vi "proiectu fara drona.vi"() -> ()   [LabVIEW 2015]
uses:
  globala.vi
  lee_3/bin/Debug/lee_3.dll
  BmpWork/lee_4/bin/Debug/lee_4.dll
panel:
  out "Numeric":dbl
  out "Image 2":T1(plugin-control)
  out "Image":T1(plugin-control)
  out "Computing Path":bool
  out "Finding START/STOP":bool
  out "Creating image from matrix":bool
  out "Started stitching":bool
  out "Started normalising and cutting":bool
  out "Curently at image":string
  out "return type 2":i32
  out "return type":i32
  in  "Numar de Poze":i32
  in  "Path to template":path
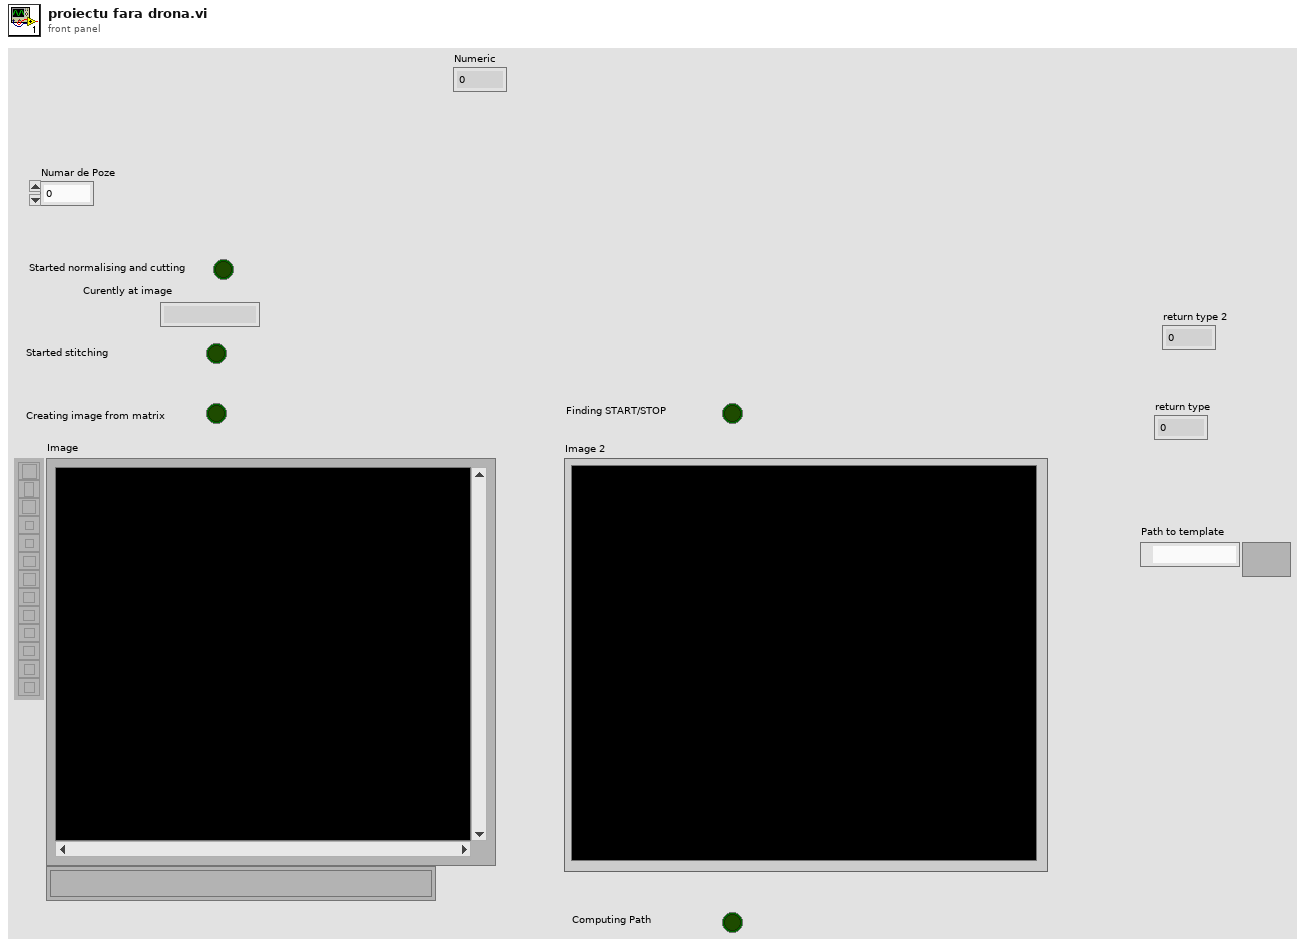
[diagram p1: front panel]
types:
  T1 = typedef "IMAQ Image.ctl" = refnum<image>
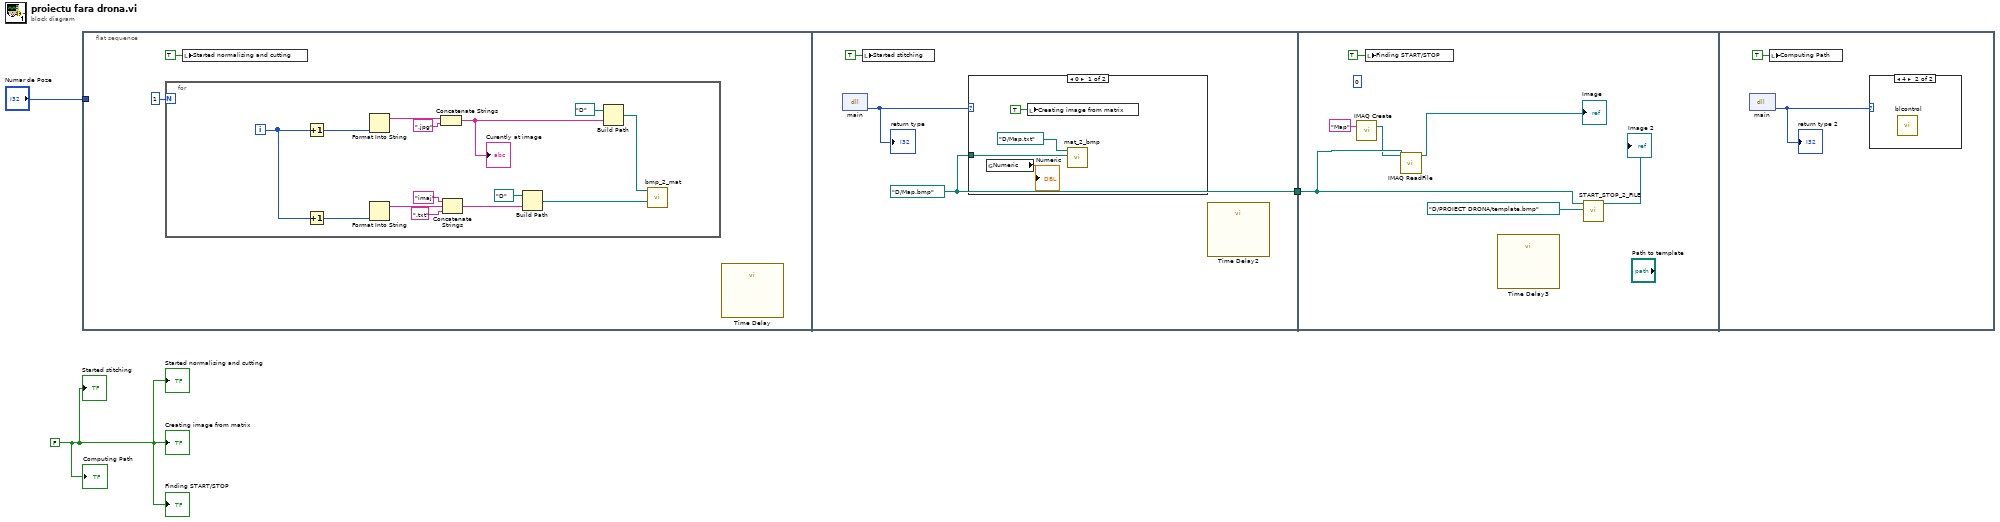
[diagram p0: block diagram]
diagram:
  w1 = FALSE
  n1 = flat-sequence {
    tunnel: "Numar de Poze" -> [_]
    tunnel: [w21] -> w3
    tunnel: w3 -> [w30]
    frame #0 {
      n2 = for {
        N: 1 -> [_]
        i -> [w8]
        n3 = Increment(x=w8) -> (x+1=w10:i32)
        n4 = Increment(x=w8) -> (x+1=w9:i32)
        n5 = Format Into String(w10) -> (resulting string=w18:string)  [unwired: 3 in, 1 out]
        n6 = Format Into String(w9) -> (resulting string=w15:string)  [unwired: 3 in, 1 out]
        n7 = Concatenate Strings(w18, ".jpg" ("string")) -> (w6:string)
        "Curently at image" <- w6
        n8 = Concatenate Strings("imaj" ("string"), w15, ".txt" ("string")) -> (w12:string)
        n9 = Build Path(base path=path "D:/", name or relative path=w12) -> (appended path=w11:path)
        n10 = Build Path(base path=path "D:/", name or relative path=w6) -> (appended path=w7:path)
        n11 = call "bmp_2_mat.vi"("Destinatia1"=w11, "Imaginea1"=w7) -> ()  [unwired: 10 in]
      }
      n12 = local write "Started normalising and cutting"(TRUE) -> ()
      n13 = call "Time Delay"() -> ()  [unwired: 11 in, 1 out]
    }
    frame #1 {
      w21 = path "D:/Map.bmp" ("Fisierul Text")
      n14 = dll-call lib="D:/PROIECT DRONA/BmpWork/lee_4/bin/Debug/lee_4.dll" fn="main"() -> ("return type"=w22:i32)  [unwired: 3 in, 2 out]
      "return type" <- w22
      n15 = local write "Started stitching"(TRUE) -> ()
      n16 = case shown="0" w22 {
        tunnel: w21 -> [w26 _]
        frame 0 {
          n17 = global read "globala.vi" "Numeric"() -> (→"Numeric":dbl)
          n18 = local write "Creating image from matrix"(TRUE) -> ()
          n19 = call "mat_2_bmp.vi"("Path"=w26, "Path 7"=path "D:/Map.txt" ("Fisierul Text")) -> ()  [unwired: 10 in]
        }
        frame 2, Default {
        }
      }
      n20 = call "Time Delay2"() -> ()  [unwired: 11 in, 1 out]
    }
    frame #2 {
      (unwired) 0 ("index")
      n21 = call "IMAQ Create"("Image Name"="Map") -> ("New Image"=w29:T1)  [unwired: 4 in, 1 out]
      n22 = local write "Finding START/STOP"(TRUE) -> ()
      n23 = call "IMAQ ReadFile"("File Path"=w30, "Image"=w29) -> ("Image Out"=→"Image":T1)  [unwired: 5 in, 4 out]
      n24 = call "Time Delay3"() -> ()  [unwired: 11 in, 1 out]
      n25 = call "START_STOP_2_FILE.vi"("Template"=path "D:/PROIECT DRONA/template.bmp" ("Path to template"), "MAP"=w30) -> ("Image"=→"Image 2":T1)  [unwired: 9 in]
    }
    frame #3 {
      n26 = dll-call lib="D:/PROIECT DRONA/lee_3/bin/Debug/lee_3.dll" fn="main"() -> ("return type"=w35:i32)  [unwired: 3 in, 2 out]
      "return type 2" <- w35
      n27 = local write "Computing Path"(TRUE) -> ()
      n28 = case shown="4" w35 {
        frame 0, Default {
        }
        frame 4 {
          n29 = call "blcontrol.vi"() -> ()  [unwired: 12 in]
        }
      }
    }
  }
  "Started normalising and cutting" <- w1
  "Creating image from matrix" <- w1
  "Finding START/STOP" <- w1
  "Computing Path" <- w1
  "Started stitching" <- w1
